vi "oa_AC DC Separation Exp (1 Channel).vi"(7 "reset? (F)":bool, 8 "points/rev":u32, 9 "averaging revolution (1)":dbl=1.0 min=0.0, 11 "even angle signal":cluster{"r0":dbl, "dr":dbl, "Y":dbl[]}={"r0"=0.0, "dr"=1.0, "Y"=[]} {"r0" format="%.2p"; "dr" format="%.2p"; "Y" format="%.2f"}) -> (0 "DC even angle signal":cluster{"r0":dbl, "dr":dbl, "Y":dbl[]}, 1 "AC even angle signal":cluster{"r0":dbl, "dr":dbl, "Y":dbl[]}, 3 "dul even angle signal":cluster{"r0":dbl, "dr":dbl, "Y":dbl[]})   [LabVIEW 2017, in "SoundVib_OAUtility.lvlib"]
uses:
  <vilib>/addons/Sound and Vibration/Order Analysis/Utility/SoundVib_OAUtility.lvlib
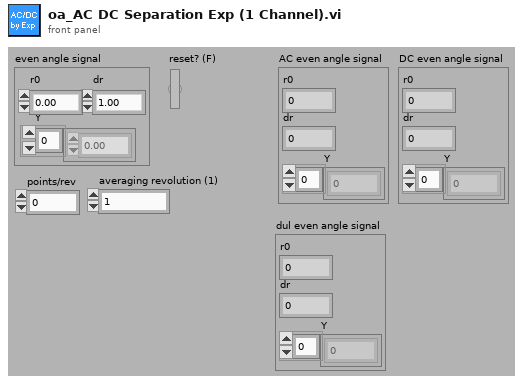
[diagram p1: front panel]
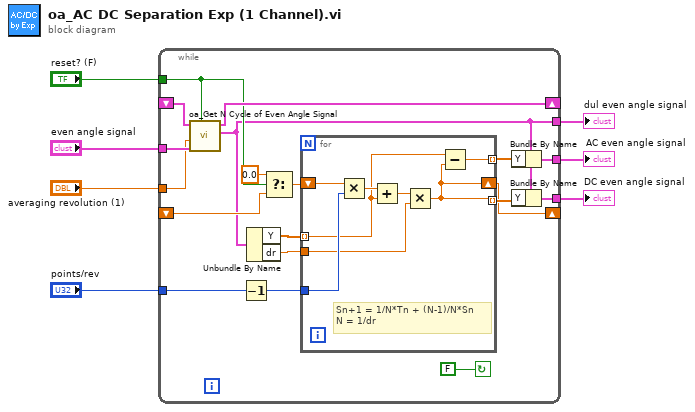
[diagram p0: block diagram]
diagram:
  n1 = while {
    tunnel: "reset? (F)" -> [w10]
    tunnel: "even angle signal" -> [w13]
    tunnel: [w19] -> w4
    tunnel: [w17] -> w3
    shift-right: [w16] -> _
    shift-left: _ -> [w15]
    tunnel: "points/rev" -> [w14]
    tunnel: [w9] -> w2
    shift-right: [w11] -> _
    shift-left: _ -> [w12]
    tunnel: "averaging revolution (1)" -> [w8]
    stop <- FALSE continue-if-true
    n2 = call <vilib>:"oa_Get N Cycle of Even Angle Signal.vi"("reset"=w10, "new even angle signal"=w13, "averaging revolution (1)"=w8, "rest even angle signal"=w12) -> ("even angle signal"=w9:cluster{"r0":dbl, "dr":dbl, "Y":dbl[]}, "rest even angle signal out"=w11:cluster{"r0":dbl, "dr":dbl, "Y":dbl[]})  [unwired: 4 in, 2 out]
    n3 = Decrement(x=w14) -> (x-1=w22:u32)
    n4 = Unbundle By Name(w9) -> ("Y"=w23:dbl[], "dr"=w21:dbl)
    n5 = Select(t=0.0, s=w10, f=w15) -> (s? t:f=w24:dbl)
    n6 = for {
      shift-right: [w27] -> w16
      shift-left: w24 -> [w34]
      tunnel: w23 -> [w29] mode=indexing
      tunnel: w22 -> [w31]
      tunnel: w21 -> [w30]
      tunnel: [w28] -> w20 mode=indexing
      tunnel: [w27] -> w18 mode=indexing
      # "Sn+1 = 1/N*Tn + (N-1)/N*Sn\nN = 1/dr"
      n7 = Multiply(x=w34, y=w31) -> (x*y=w33:dbl)
      n8 = Add(x=w33, y=w29) -> (x+y=w32:dbl)
      n9 = Multiply(x=w32, y=w30) -> (x*y=w27:dbl)
      n10 = Subtract(x=w29, y=w27) -> (x-y=w28:dbl)
    }
    n11 = Bundle By Name(cluster=w9, "Y"=w20) -> (w19:cluster{"r0":dbl, "dr":dbl, "Y":dbl[]})
    n12 = Bundle By Name(cluster=w9, "Y"=w18) -> (w17:cluster{"r0":dbl, "dr":dbl, "Y":dbl[]})
  }
  "AC even angle signal" <- w4
  "DC even angle signal" <- w3
  "dul even angle signal" <- w2
